vi "FindMutationHistoryIndex.vi"(9 "Old Name Index":u8, 10 "Library Version":T1, 11 "Mutation History":T2=[{"Library Version"={"Major"=1, "Minor"=0, "Fix"=0, "Build"=0}, "Old Name Index"=1, "Class Default Data"=variant, "Cluster Order Map"=[], "Parent Name"="", "Parent Path"=path "", "LabVIEW Version"=0, "User Comments"="", "Mutation Flags"=0, "Parent Old Name Index"=0, "Parent Levels Added"=0, "Parent Levels Removed"=0}, {"Library Version"={"Major"=1, "Minor"=0, "Fix"=1, "Build"=1}, "Old Name Index"=1, "Class Default Data"=variant, "Cluster Order Map"=[], "Parent Name"="", "Parent Path"=path "", "LabVIEW Version"=0, "User Comments"="", "Mutation Flags"=0, "Parent Old Name Index"=0, "Parent Levels Added"=0, "Parent Levels Removed"=0}, {"Library Version"={"Major"=2, "Minor"=0, "Fix"=0, "Build"=2}, "Old Name Index"=0, "Class Default Data"=variant, "Cluster Order Map"=[], "Parent Name"="", "Parent Path"=path "", "LabVIEW Version"=0, "User Comments"="", "Mutation Flags"=0, "Parent Old Name Index"=0, "Parent Levels Added"=0, "Parent Levels Removed"=0}, {"Library Version"={"Major"=2, "Minor"=0, "Fix"=1, "Build"=3}, "Old Name Index"=0, "Class Default Data"=variant, "Cluster Order Map"=[], "Parent Name"="", "Parent Path"=path "", "LabVIEW Version"=0, "User Comments"="", "Mutation Flags"=0, "Parent Old Name Index"=0, "Parent Levels Added"=0, "Parent Levels Removed"=0}, {"Library Version"={"Major"=2, "Minor"=1, "Fix"=0, "Build"=4}, "Old Name Index"=0, "Class Default Data"=variant, "Cluster Order Map"=[], "Parent Name"="", "Parent Path"=path "", "LabVIEW Version"=0, "User Comments"="", "Mutation Flags"=0, "Parent Old Name Index"=0, "Parent Levels Added"=0, "Parent Levels Removed"=0}] {"LabVIEW Version" format="%.0x"}) -> (2 "Found?":bool, 3 "Index":i32)   [LabVIEW 2019, in "BlueSerializationProviderShared.lvlib"]
uses:
  BlueSerializationProviderShared.lvlib
  <vilib>/Utility/EditLVLibs/LVClass/Mutation History.ctl
  <vilib>/Utility/EditLVLibs/LVClass/Mutation Record.ctl
  <vilib>/Utility/EditLVLibs/LibVersion.ctl
  <vilib>/Utility/EditLVLibs/Edit LVLibs.lvlib
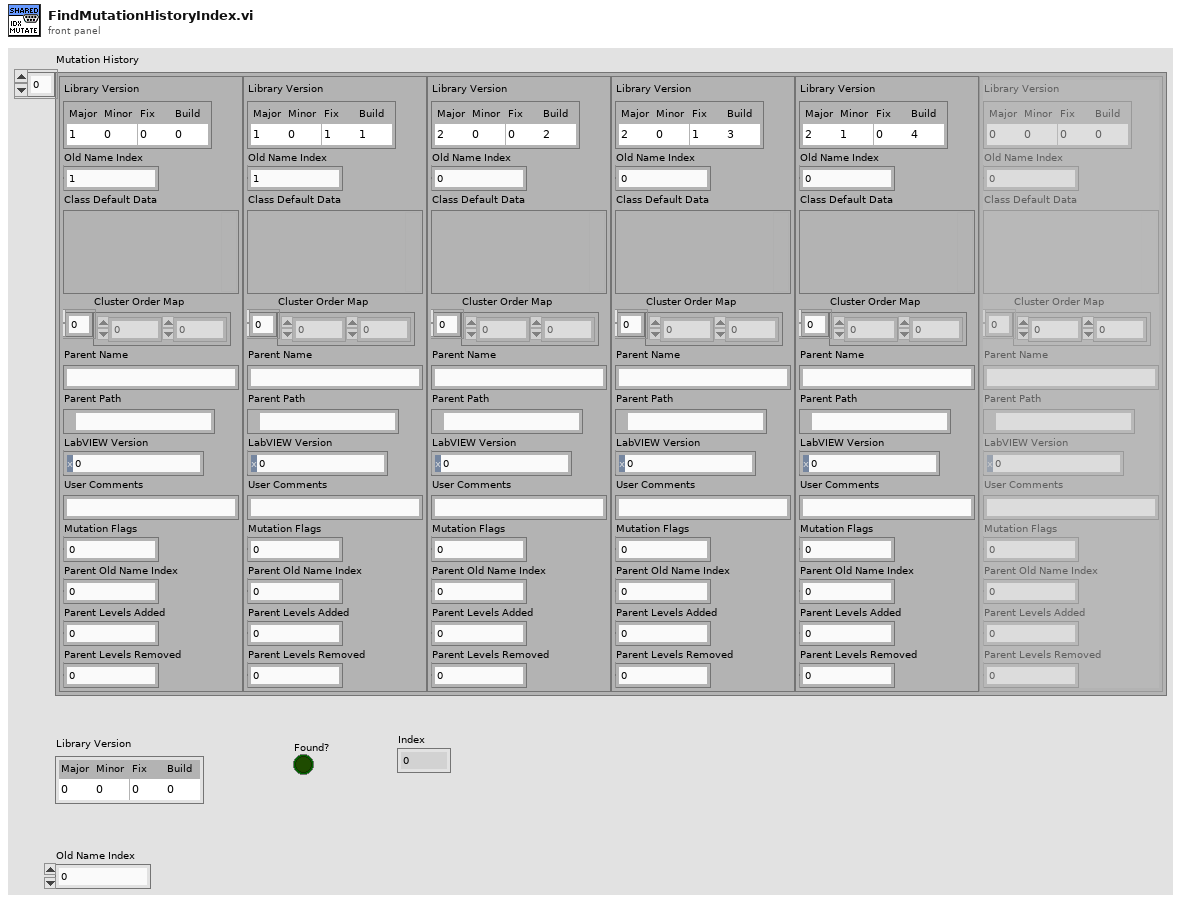
[diagram p1: front panel]
types:
  T1 = typedef "Edit LVLibs.lvlib/LibVersion.ctl" = cluster{"Major":u16, "Minor":u16, "Fix":u16, "Build":u16}
  T2 = typedef "Edit LVLibs.lvlib/Mutation History.ctl" = T3[]
  T3 = typedef "Edit LVLibs.lvlib/Mutation Record.ctl" = cluster{"Library Version":T1, "Old Name Index":u8, "Class Default Data":variant, "Cluster Order Map":u32[], "Parent Name":string, "Parent Path":path, "LabVIEW Version":u32, "User Comments":string, "Mutation Flags":u8, "Parent Old Name Index":u8, "Parent Levels Added":u16, "Parent Levels Removed":u16}
  T4 = cluster{"Library Version":T1, "Old Name Index":u8}
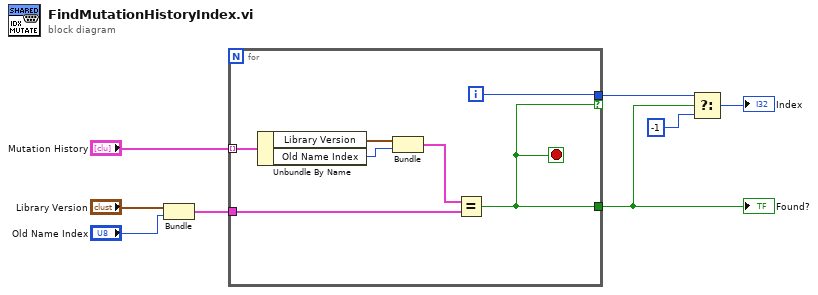
[diagram p0: block diagram]
diagram:
  n1 = Bundle("Library Version"="Library Version", "Old Name Index"="Old Name Index") -> (w6:T4)  [unwired: 1 in]
  n2 = for {
    tunnel: "Mutation History" -> [w15] mode=indexing
    tunnel: w6 -> [w11]
    tunnel: [w10] -> w3 if=w9
    tunnel: [w9] -> w4
    i -> [w10]
    stop <- w9 stop-if-true
    n3 = Unbundle By Name(w15) -> ("Library Version"=w14:T1, "Old Name Index"=w13:u8)
    n4 = Bundle("Library Version"=w14, "Old Name Index"=w13) -> (w12:T4)  [unwired: 1 in]
    n5 = Equal?(x=w12, y=w11) -> (x = y?=w9:bool)
  }
  "Found?" <- w4
  n6 = Select(t=w3, s=w4, f=-1) -> (s? t:f=→"Index":i32)
